vi "oax_Read Tacho and Vibration Data (Digital Tacho).vi"(0 "refnum":refnum<file>, 1 "reset? (T)":bool=TRUE, 11 "error in (no error)":errorcluster) -> (3 "pulse / rev":i32, 4 "refnum out":refnum<file>, 6 "waveform data":waveform(dbl)[](array[waveform]), 8 "digital tacho info":T4={"tacho counts"=[], "counter timebase [Hz]"=20000000.0, "counter task type"=enum."event counting", "counter digit (32)"=32}, 10 "channel info":T1[](array[typedef]) {"pregain" format="%.2f"; "weighting filter" items=["Linear", "A-weighting", "B-weighting", "C-weighting", "ITU-R 468-4", "Dolby", "CCITT", "C-message", "Wb", "Wc", "Wd", "We", "Wf", "Wh", "Wj", "Wk", "Wm", "AES17 20 kHz lowpass", "AES17 40 kHz lowpass", "AES17 20 kHz highpass", "AES17 40 kHz highpass"]; "dB reference" format="%^.1e"; "engineering units" items=["custom..."=0, "V"=1, "A"=21, "C"=30, "pC"=31, "s"=32, "-"=29, "Pa"=2, "N"=20, "g"=3, "m/s^2"=4, "m/s"=5, "m"=6, "mm/s"=12, "mm"=13, "micron/s"=14, "micron"=15, "in/s^2"=7, "in/s"=8, "in"=9, "mil/s"=10, "mil"=11, "rad/s^2"=16, "rad/s"=17, "rad"=18, "deg/s^2"=26, "deg/s"=27, "deg"=28, "RPM"=22, "cycle/s^2"=23, "Hz"=24, "cycle"=25, "strain"=19]; "sensor sensitivity" format="%#_5f"}, 14 "channel name":string[](array[string]), 15 "error out":errorcluster)   [LabVIEW 2017]
uses:
  <vilib>/addons/Sound and Vibration/Order Analysis/Tach Process/SubVIs/digital tach info.ctl
  <vilib>/addons/_NISVFA/_Shared subVIs/Controls/svc_Channel Info.ctl
  <vilib>/addons/_NISVFA/_Shared subVIs/Controls/svc_Engineering Units Text Ring.ctl
  <vilib>/addons/_NISVFA/_Shared subVIs/Controls/svc_Weighting Filter Text Ring.ctl
  <vilib>/Waveform/WDTOps.llb/WDT Append Waveforms DBL.vi
  <vilib>/addons/Sound and Vibration/Order Analysis/Tach Process/SoundVib_TachProcess.lvlib
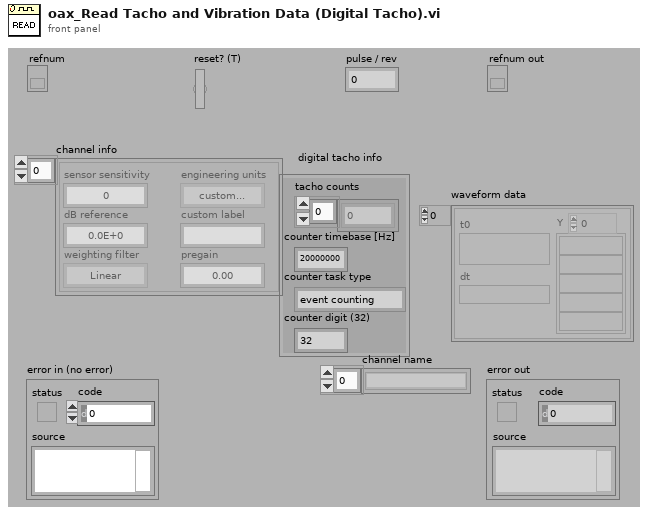
[diagram p1: front panel]
types:
  T1 = typedef "svc_Channel Info.ctl" = cluster{"sensor sensitivity":dbl, "engineering units":T2, "dB reference":dbl, "custom label":string, "weighting filter":T3, "pregain":dbl}
  T2 = typedef "svc_Engineering Units Text Ring.ctl" = u16
  T3 = typedef "svc_Weighting Filter Text Ring.ctl" = u16
  T4 = typedef "SoundVib_TachProcess.lvlib/digital tach info.ctl" = cluster{"tacho counts":i64[], "counter timebase [Hz]":dbl, "counter task type":enum16{"period measurement", "event counting"}, "counter digit (32)":i32}
  T5 = cluster{"digital tacho info":cluster{"tacho counts":i32[], "counter timebase [Hz]":dbl, "counter task type":enum16{"period measurement", "event counting"}, "counter digit (32)":i32}, "waveform data":waveform(dbl)[]}
  T6 = cluster{"tacho counts":i32[], "counter timebase [Hz]":dbl, "counter task type":enum16{"period measurement", "event counting"}, "counter digit (32)":i32}
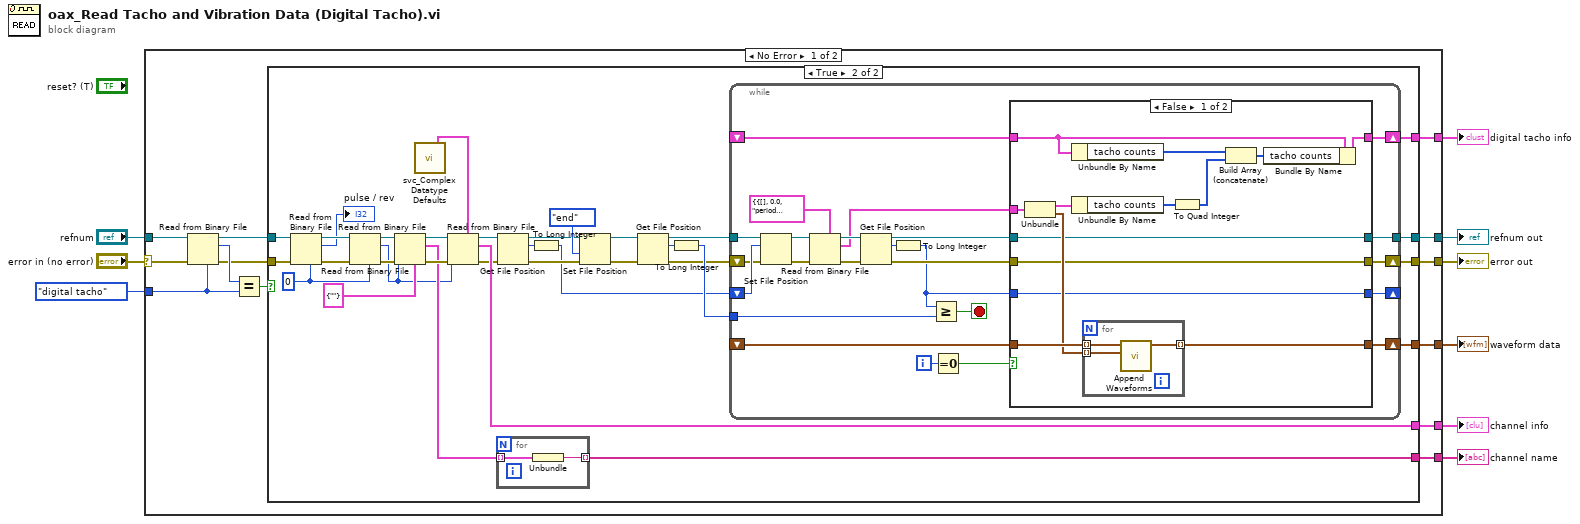
[diagram p0: block diagram]
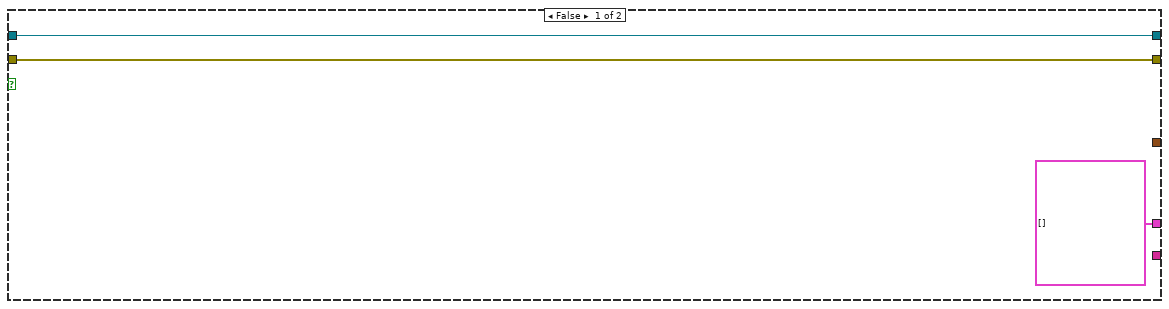
[diagram p2: hidden frame]
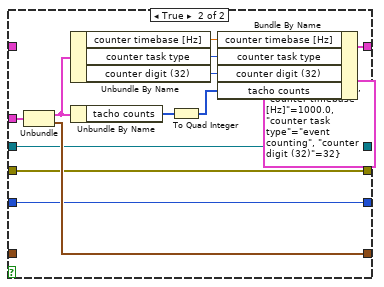
[diagram p3: hidden frame]
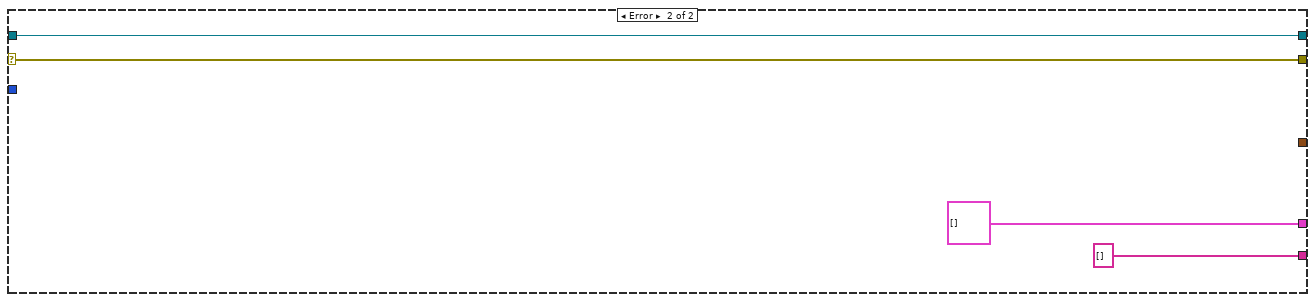
[diagram p4: hidden frame]
diagram:
  n1 = case shown="No Error" "error in (no error)" {
    selector: "error in (no error)" -> [w19 w118]
    tunnel: [w13 w118] -> w8
    tunnel: "refnum" -> [w22 w117]
    tunnel: [w14 w117] -> w6
    tunnel: [w16 T1[] []] -> w5
    tunnel: [w15 string[] []] -> w4
    tunnel: [w12 _] -> w3
    tunnel: [w11 _] -> w2
    tunnel: enum16{"analog tacho", "digital tacho"}."digital tacho" -> [w10 _]
    frame No Error {
      n2 = Read from Binary File(5:w10, 8:w19, 11:w22) -> (0:w17:errorcluster, 2:w21:enum16{"analog tacho", "digital tacho"}, 3:w18:refnum<file>)  [unwired: 3 in, 1 out]
      n3 = Equal?(x=w21, y=w10) -> (x = y?=w20:bool)
      n4 = case shown="True" w20 {
        tunnel: w18 -> [w25 w57]
        tunnel: w17 -> [w24 w58]
        tunnel: [T1[] [] w46] -> w16
        tunnel: [_ w50] -> w15
        tunnel: [w25 w41] -> w14
        tunnel: [w24 w40] -> w13
        tunnel: [_ w37] -> w12
        tunnel: [_ w39] -> w11
        frame False {
        }
        frame True {
          w45 = 0
          n5 = Read from Binary File(5:w45, 8:w58, 11:w57) -> (0:w54:errorcluster, 2:→"pulse / rev":i32, 3:w52:refnum<file>)  [unwired: 3 in, 1 out]
          n6 = Read from Binary File(5:w45, 8:w54, 11:w52) -> (0:w53:errorcluster, 2:w36:i32, 3:w51:refnum<file>)  [unwired: 3 in, 1 out]
          n7 = Read from Binary File(5:cluster{"ch0 string":string} {"ch0 string"=""}, 8:w53, 10:w36, 11:w51) -> (0:w56:errorcluster, 2:w47:cluster{"ch0 string":string}[], 3:w55:refnum<file>)  [unwired: 2 in, 1 out]
          n8 = call <vilib>:"svc_Complex Datatype Defaults.vi"() -> ("channel info"=w26:T1)  [unwired: 11 in, 8 out]
          n9 = Read from Binary File(5:w26, 8:w56, 10:w36, 11:w55) -> (0:w28:errorcluster, 2:w46:T1[], 3:w29:refnum<file>)  [unwired: 2 in, 1 out]
          n10 = for {
            tunnel: w47 -> [w114] mode=indexing
            tunnel: [w113] -> w50 mode=indexing
            n11 = Unbundle(w114) -> ("ch0 string"=w113:string)
          }
          n12 = Get File Position(4:w28, 7:w29) -> (0:w35:errorcluster, 2:w27:i64, 3:w34:refnum<file>)
          n13 = To Long Integer(number=w27) -> (32bit integer=w33:i32)
          n14 = Set File Position(refnum=w34, from (0:start)=enum16{"start", "end", "current"}."end" ("pos mode (0:2)"), error in=w35) -> (refnum out=w32:refnum<file>, error out=w31:errorcluster)  [unwired: 1 in]
          n15 = Get File Position(4:w31, 7:w32) -> (0:w38:errorcluster, 2:w30:i64, 3:w43:refnum<file>)
          n16 = To Long Integer(number=w30) -> (32bit integer=w42:i32)
          n17 = while {
            tunnel: w43 -> [w82]
            shift-right: [w60] -> _
            shift-left: w33 -> [w81]
            tunnel: w42 -> [w80]
            tunnel: [w64] -> w41
            shift-right: [w68] -> w39
            shift-left: _ -> [w67]
            shift-right: [w63] -> w40
            shift-left: w38 -> [w77]
            shift-right: [w71] -> w37
            shift-left: _ -> [w69]
            i -> [w78]
            stop <- w79 stop-if-true
            n18 = Set File Position(offset (in bytes) (0)=w81, refnum=w82, error in=w77) -> (refnum out=w76:refnum<file>, error out=w75:errorcluster)  [unwired: 1 in]
            n19 = Read from Binary File(5:T5 {"digital tacho info"={"tacho counts"=[], "counter timebase [Hz]"=0.0, "counter task type"=enum."period measurement", "counter digit (32)"=0}, "waveform data"=[]} ("output cluster"), 8:w75, 11:w76) -> (0:w73:errorcluster, 2:w66:T5, 3:w74:refnum<file>)  [unwired: 3 in, 1 out]
            n20 = Get File Position(4:w73, 7:w74) -> (0:w62:errorcluster, 2:w72:i64, 3:w65:refnum<file>)
            n21 = To Long Integer(number=w72) -> (32bit integer=w61:i32)
            n22 = Greater Or Equal?(x=w61, y=w80) -> (x >= y?=w79:bool)
            n23 = Equal To 0?(x=w78) -> (x = 0?=w70:bool)
            n24 = case shown="False" w70 {
              tunnel: [w93 w110] -> w71
              tunnel: w69 -> [w91 _]
              tunnel: [w90 w104] -> w68
              tunnel: w67 -> [w89 _]
              tunnel: w66 -> [w88 w106]
              tunnel: w65 -> [w85 w103]
              tunnel: [w85 w103] -> w64
              tunnel: [w84 w102] -> w63
              tunnel: w62 -> [w84 w102]
              tunnel: w61 -> [w83 w101]
              tunnel: [w83 w101] -> w60
              frame False {
                n25 = Unbundle(w88) -> ("digital tacho info"=w87:T6, "waveform data"=w86:waveform(dbl)[])
                n26 = Unbundle By Name(w91) -> ("tacho counts"=w95:i64[])
                n27 = Unbundle By Name(w87) -> ("tacho counts"=w96:i32[])
                n28 = for {
                  tunnel: w86 -> [w99] mode=indexing
                  tunnel: [w98] -> w90 mode=indexing
                  tunnel: w89 -> [w97] mode=indexing
                  n29 = call-poly <vilib>:"Append Waveforms.vi"("waveform B"=w99, "waveform A"=w97) -> ("waveform out"=w98:waveform(dbl))  [unwired: 8 in, 1 out]
                }
                n30 = To Quad Integer(1:w96) -> (0:w94:i64[])
                n31 = Build Array (concatenate)(w95, w94) -> (w92:i64[])
                n32 = Bundle By Name(cluster=w91, "tacho counts"=w92) -> (w93:T4)
              }
              frame True {
                n33 = Unbundle(w106) -> ("digital tacho info"=w105:T6, "waveform data"=w104:waveform(dbl)[])
                n34 = Unbundle By Name(w105) -> ("counter timebase [Hz]"=w109:dbl, "counter task type"=w108:enum16{"period measurement", "event counting"}, "counter digit (32)"=w107:i32)
                n35 = Unbundle By Name(w105) -> ("tacho counts"=w112:i32[])
                n36 = To Quad Integer(1:w112) -> (0:w111:i64[])
                n37 = Bundle By Name(cluster=T4 {"tacho counts"=[], "counter timebase [Hz]"=1000.0, "counter task type"=enum."event counting", "counter digit (32)"=32} ("t"), "counter timebase [Hz]"=w109, "counter task type"=w108, "counter digit (32)"=w107, "tacho counts"=w111) -> (w110:T4)
              }
            }
          }
        }
      }
    }
    frame Error {
    }
  }
  "error out" <- w8
  "waveform data" <- w2
  "digital tacho info" <- w3
  "refnum out" <- w6
  "channel name" <- w4
  "channel info" <- w5
